vi "LabVIEW GUI - single threshold.vi"() -> ()   [LabVIEW 2021]
uses:
  <vilib>/Instr/_visa.llb/VISA Configure Serial Port (Instr).vi
panel:
  out "Thermometer":dbl(slide) scale=0.0..40.0
  out "LED":bool
  out "Buffer":string
  out "Waveform Chart":cluster{dbl, dbl, i32}(graph)
  in  "stop":bool
  in  "Arduino COM Port":refnum<visa-resource-name>="COM3"
  # "Thermistor-based Thermostat with single threshold"
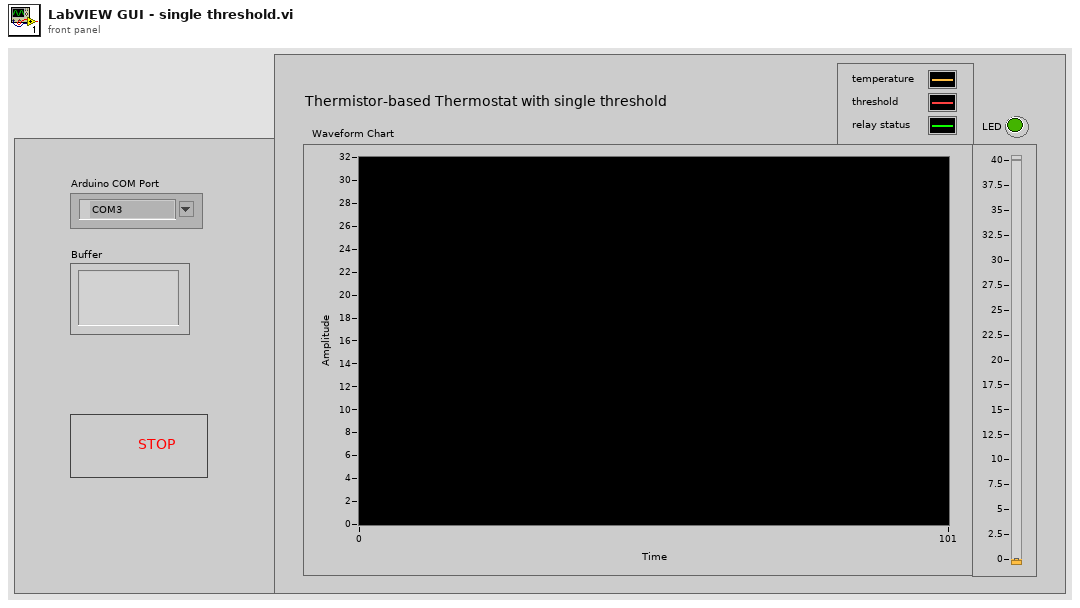
[diagram p1: front panel]
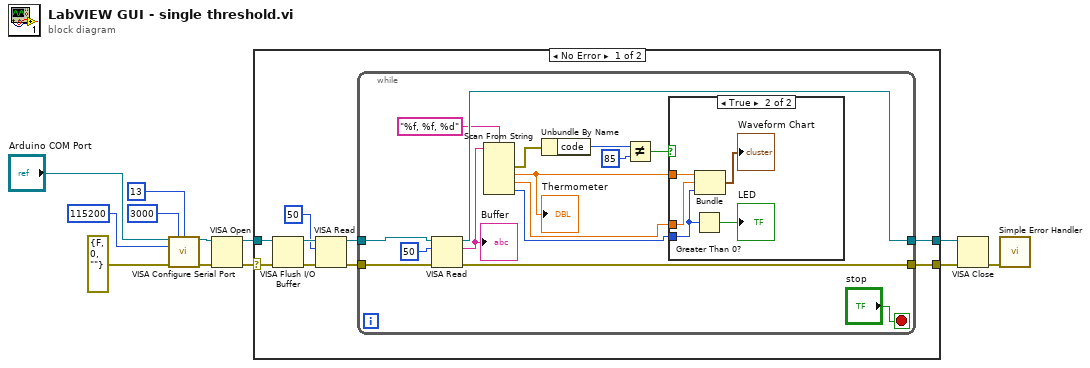
[diagram p0: block diagram]
diagram:
  n1 = call-poly "VISA Configure Serial Port"("VISA resource name"="Arduino COM Port", "timeout (10sec)"=u32 3000, "termination char\n(0xA = '\\n' = LF)"=u8 13 ("termination char\n(0xA = '\\n' = LF)"), "baud rate (9600)"=u32 115200, "error in (no error)"=errorcluster {"status"=FALSE, "code"=0, "source"=""}) -> ("VISA resource name out"=w7:refnum<visa-resource-name>, "error out"=w8:errorcluster)  [unwired: 9 in]
  n2 = VISA Open(error in (no error)=w8, VISA resource name=w7) -> (VISA resource name=w6:refnum<visa-resource-name>, error out=w5:errorcluster)  [unwired: 3 in]
  n3 = case shown="No Error" w5 {
    selector: w5 -> [w15 w42]
    tunnel: w6 -> [w19 w43]
    tunnel: [w14 w42] -> w3
    tunnel: [w13 w43] -> w2
    frame No Error {
      n4 = VISA Flush I/O Buffer(VISA resource name=w19, error in (no error)=w15) -> (VISA resource name out=w18:refnum<visa-resource-name>, error out=w17:errorcluster)  [unwired: 1 in]
      n5 = VISA Read(VISA resource name=w18, byte count=u32 50, error in (no error)=w17) -> (VISA resource name out=w20:refnum<visa-resource-name>, error out=w21:errorcluster)  [unwired: 2 out]
      n6 = while {
        tunnel: w20 -> [w34]
        tunnel: [w33] -> w13
        tunnel: w21 -> [w36]
        tunnel: [w35] -> w14
        stop <- "stop" stop-if-true
        n7 = VISA Read(VISA resource name=w34, byte count=u32 50, error in (no error)=w36) -> (VISA resource name out=w33:refnum<visa-resource-name>, read buffer=w23:string, error out=w35:errorcluster)  [unwired: 1 out]
        "Buffer" <- w23
        n8 = Scan From String(format string="%f, %f, %d", input string=w23) -> (error out=w27:errorcluster, output 1=w22:dbl, output 2=w29:dbl, output 3=w28:i32)  [unwired: 5 in, 2 out]
        "Thermometer" <- w22
        n9 = Unbundle By Name(w27) -> ("code"=w26:i32)
        n10 = Not Equal?(x=w26, y=85) -> (x != y?=w24:bool)
        n11 = case shown="True" w24 {
          tunnel: w22 -> [_ w41]
          tunnel: w29 -> [_ w40]
          tunnel: w28 -> [_ w38]
          frame False {
          }
          frame True {
            n12 = Greater Than 0?(x=w38) -> (x > 0?=→"LED":bool)
            n13 = Bundle("Thermometer"=w41, w40, w38) -> (→"Waveform Chart":cluster{"Thermometer":dbl, dbl, i32})  [unwired: 1 in]
          }
        }
      }
    }
    frame Error {
    }
  }
  n14 = VISA Close(VISA resource name=w2, error in (no error)=w3) -> (error out=w1:errorcluster)
  n15 = call <vilib>:"Simple Error Handler.vi"("error in (no error)"=w1) -> ()  [unwired: 4 in, 5 out]
